vi "Database Editing UI.vi"() -> ()   [LabVIEW 2016]
doc: "UI for editing the database configuration files directly"
uses:
  Car Wash Controller/Controls/Steps.ctl
  Car Wash Controller/Controls/Stations.ctl
panel:
  in  "Stop Button":bool
  in  "Save Button":bool
  in  "Open Button":bool
  in  "Records":T3(array[cluster])
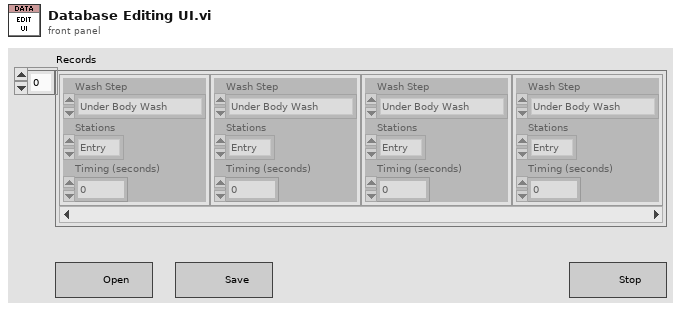
[diagram p1: front panel]
types:
  T1 = typedef "Steps.ctl" = enum16{"Under Body Wash", "Bug Remover", "Pre-Soak", "High Pressure Wash", "Low Pressure Wax", "Spot Free Rinse", "Tire Shine Foam", "Air Dry"}
  T2 = typedef "Stations.ctl" = enum16{"Entry", "Station 1", "Station 2", "Station 3", "Exit"}
  T3 = cluster{"Wash Step":T1, "Stations":T2, "Timing (seconds)":u32}[]
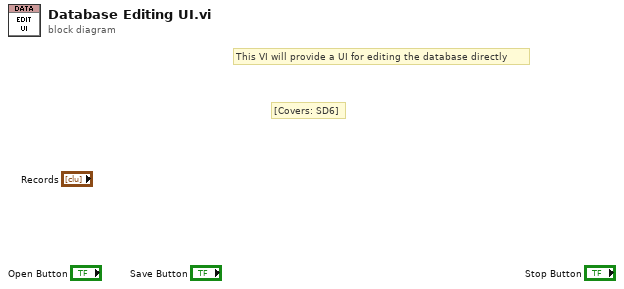
[diagram p0: block diagram]
diagram:
  # "[Covers: SD6]"
  # "This VI will provide a UI for editing the database directly"
